vi "init.vi"(8 "error in":errorcluster, 10 "TBM module configuration in":refnum<class "TBM module configuration.lvclass">, 11 "Tag Bus Web Interface runtime in":refnum<class "Tag Bus Web Interface runtime.lvclass">) -> (0 "error out":errorcluster, 1 "data allocations":T1, 2 "execution settings":T4, 3 "Tag Bus Web Interface runtime out":refnum<class "Tag Bus Web Interface runtime.lvclass">)   [LabVIEW 2013, in "Tag Bus Web Interface runtime.lvclass"]
doc: "Provides an interface for initializing a module at runtime. While this interface performs no operations, a child should provide an override which may open any necessary references or sessions, allocate necessary memory, and perform any final configuration validataion before providing the full configuration <b>execution data</b> to the calling process."
uses:
  Tag Bus Web Interface runtime.lvclass
  <vilib>/NI/Tag Bus Module Framework/module configuration/TBM module configuration.lvclass
  <vilib>/NI/Tag Bus Module Framework/runtime/execution settings.ctl
  <vilib>/NI/Tag Bus Module Framework/channel/data tables.ctl
  <vilib>/NI/Tag Bus/dictionary/data dictionary.lvclass
  <vilib>/NI/Tag Bus/dictionary table pair.ctl
  <vilib>/NI/Tag Bus/table/data table.ctl
  configuration/Tag Bus Web Interface configuration.lvclass
  Tag Bus Web Interface runtime.lvclass/Tag Bus Web Interface runtime.ctl
  <vilib>/NI/Tag Bus Module Framework/channel/TBM channel.lvclass
  <vilib>/NI/Tag Bus Module Framework/runtime/TBM module execution interface.lvclass
  <vilib>/NI/Tag Bus/tag bus.lvlib
  <vilib>/NI/Tag Bus/table/data table.lvlib
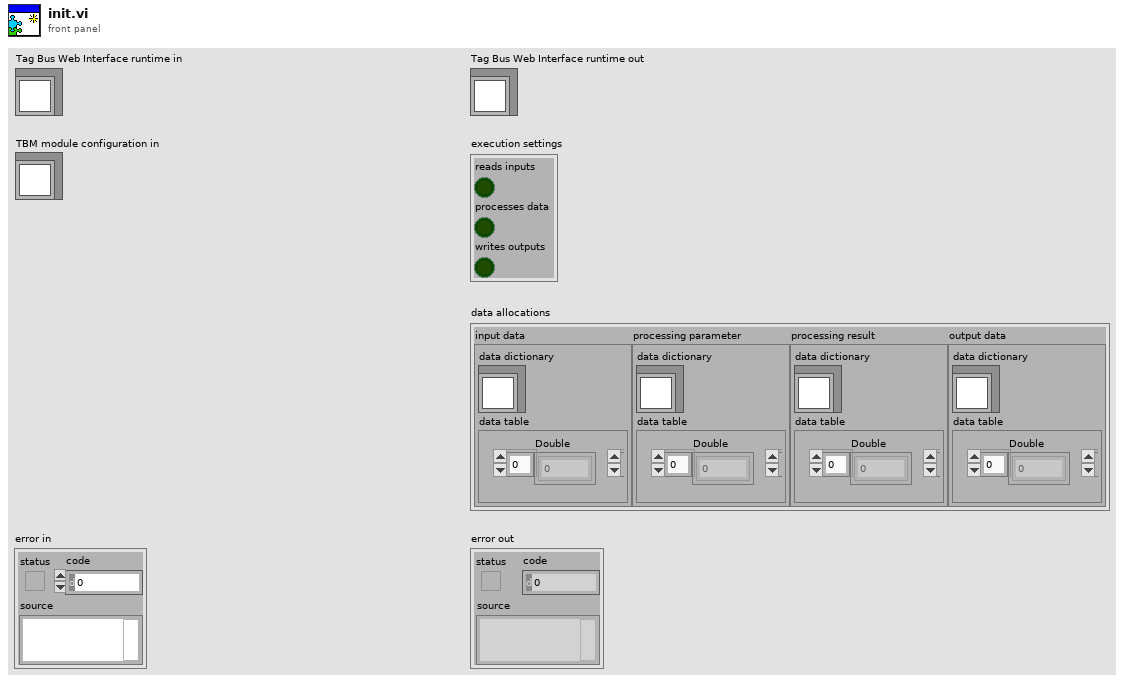
[diagram p1: front panel]
types:
  T1 = typedef "TBM channel.lvclass/data tables.ctl" = cluster{"input data":T2, "processing parameter":T2, "processing result":T2, "output data":T2}
  T2 = typedef "tag bus.lvlib/dictionary table pair.ctl" = cluster{"data dictionary":refnum<class "data dictionary.lvclass">, "data table":T3}
  T3 = typedef "tag bus.lvlib/data table.lvlib/data table.ctl" = cluster{"Double":dbl[], "Single":sgl[], "I64":i64[], "I32":i32[], "I16":i16[], "I8":i8[], "U64":u64[], "U32":u32[], "U16":u16[], "U8":u8[], "Boolean":bool[], "String":string[], "Array of Double":cluster{"DBL Array":dbl[]}[], "Array of Single":cluster{"SGL Array":sgl[]}[], "Array of I64":cluster{"I64 Array":i64[]}[], "Array of I32":cluster{"I32 Array":i32[]}[], "Array of I16":cluster{"I16 Array":i16[]}[], "Array of I8":cluster{"I8 Array":i8[]}[], "Array of U64":cluster{"U64 Array":u64[]}[], "Array of U32":cluster{"U32 Array":u32[]}[], "Array of U16":cluster{"U16 Array":u16[]}[], "Array of U8":cluster{"U8 Array":u8[]}[], "Array of Boolean":cluster{"Boolean Array":bool[]}[], "Array of String":cluster{"String Array":string[]}[]}
  T4 = typedef "TBM module execution interface.lvclass/execution settings.ctl" = cluster{"reads inputs":bool, "processes data":bool, "writes outputs":bool}
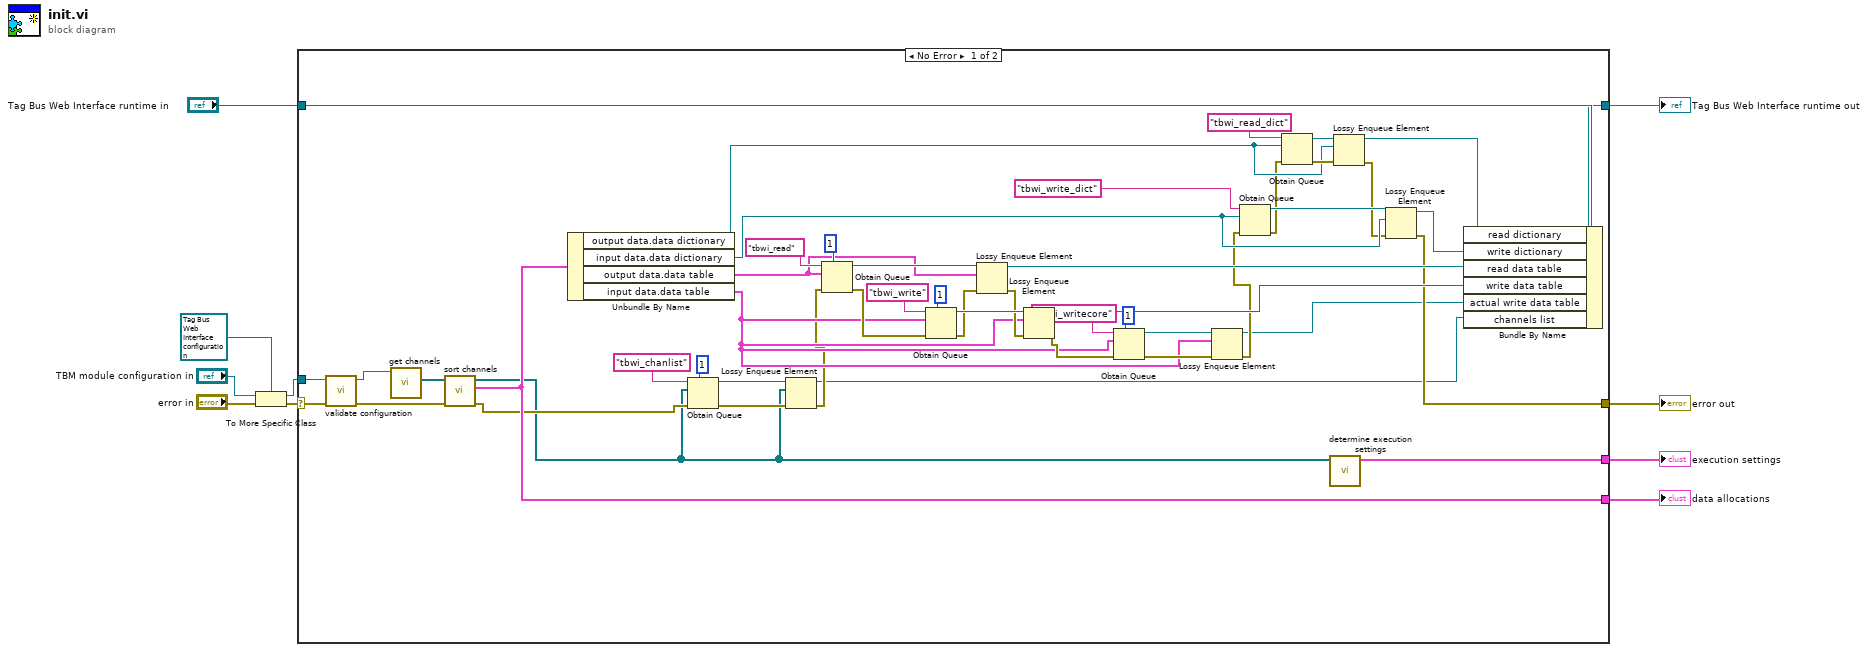
[diagram p0: block diagram]
diagram:
  n1 = To More Specific Class(target class=refnum<class "Tag Bus Web Interface configuration.lvclass"> refnum ("Synchronous module configuration"), reference="TBM module configuration in", error in="error in") -> (specific class reference=w9:refnum<class "Tag Bus Web Interface configuration.lvclass">, error out=w10:errorcluster)
  n2 = case shown="No Error" w10 {
    selector: w10 -> [w57 w60]
    tunnel: w9 -> [w56 _]
    tunnel: "Tag Bus Web Interface runtime in" -> [w29 w61]
    tunnel: [w28 w61] -> w4
    tunnel: [w27 w60] -> w3
    tunnel: [w30 _] -> w1
    tunnel: [w59 _] -> w2
    frame No Error {
      n3 = call-dynamic "validate configuration.vi"("error in"=w57, "Tag Bus Web Interface configuration in"=w56) -> ("error out"=w58:errorcluster, "Tag Bus Web Interface configuration out"=w55:refnum<class "Tag Bus Web Interface configuration.lvclass">)  [unwired: 8 in]
      n4 = call-dynamic "get channels.vi"("Tag Bus Web Interface configuration in"=w55) -> ("channels"=w54:refnum<class "TBM channel.lvclass">[])  [unwired: 9 in, 1 out]
      n5 = call <vilib>:"sort channels.vi"("error in"=w58, "channels in"=w54) -> ("error out"=w14:errorcluster, "data allocations"=w30:T1, "channels out"=w13:refnum<class "TBM channel.lvclass">[])  [unwired: 7 in]
      n6 = Unbundle By Name(w30) -> ("output data.data dictionary"=w40:refnum<class "data dictionary.lvclass">, "input data.data dictionary"=w38:refnum<class "data dictionary.lvclass">, "output data.data table"=w48:T3, "input data.data table"=w20:T3)
      n7 = Obtain Queue(max queue size (-1, unlimited)=1, name (unnamed)="tbwi_chanlist", element data type=w13, error in (no error)=w14) -> (queue out=w17:refnum<queue>, error out=w16:errorcluster)  [unwired: 1 in, 1 out]
      n8 = Lossy Enqueue Element(queue=w17, element=w13, error in (no error)=w16) -> (queue out=w11:refnum<queue>, error out=w12:errorcluster)  [unwired: 2 out]
      n9 = Obtain Queue(max queue size (-1, unlimited)=1, name (unnamed)="tbwi_read", element data type=w48, error in (no error)=w12) -> (queue out=w49:refnum<queue>, error out=w50:errorcluster)  [unwired: 1 in, 1 out]
      n10 = Obtain Queue(max queue size (-1, unlimited)=1, name (unnamed)="tbwi_write", element data type=w20, error in (no error)=w50) -> (queue out=w47:refnum<queue>, error out=w46:errorcluster)  [unwired: 1 in, 1 out]
      n11 = Lossy Enqueue Element(queue=w49, element=w48, error in (no error)=w46) -> (queue out=w33:refnum<queue>, error out=w45:errorcluster)  [unwired: 2 out]
      n12 = Lossy Enqueue Element(queue=w47, element=w20, error in (no error)=w45) -> (queue out=w32:refnum<queue>, error out=w22:errorcluster)  [unwired: 2 out]
      n13 = Obtain Queue(max queue size (-1, unlimited)=1, name (unnamed)="tbwi_writecore", element data type=w20, error in (no error)=w22) -> (queue out=w24:refnum<queue>, error out=w25:errorcluster)  [unwired: 1 in, 1 out]
      n14 = Lossy Enqueue Element(queue=w24, element=w20, error in (no error)=w25) -> (queue out=w19:refnum<queue>, error out=w21:errorcluster)  [unwired: 2 out]
      n15 = Obtain Queue(name (unnamed)="tbwi_write_dict", element data type=w38, error in (no error)=w21) -> (queue out=w39:refnum<queue>, error out=w37:errorcluster)  [unwired: 2 in, 1 out]
      n16 = Obtain Queue(name (unnamed)="tbwi_read_dict", element data type=w40, error in (no error)=w37) -> (queue out=w41:refnum<queue>, error out=w42:errorcluster)  [unwired: 2 in, 1 out]
      n17 = call <vilib>:"determine execution settings.vi"("channels"=w13) -> ("execution settings"=w59:T4)  [unwired: 10 in]
      n18 = Lossy Enqueue Element(queue=w41, element=w40, error in (no error)=w42) -> (queue out=w35:refnum<queue>, error out=w36:errorcluster)  [unwired: 2 out]
      n19 = Lossy Enqueue Element(queue=w39, element=w38, error in (no error)=w36) -> (queue out=w34:refnum<queue>, error out=w27:errorcluster)  [unwired: 2 out]
      n20 = Bundle By Name(cluster=w29, "read dictionary"=w35, "write dictionary"=w34, "read data table"=w33, "write data table"=w32, "actual write data table"=w19, "channels list"=w11) -> (w28:refnum<class "Tag Bus Web Interface runtime.lvclass">)
    }
    frame Error {
    }
  }
  "error out" <- w3
  "Tag Bus Web Interface runtime out" <- w4
  "execution settings" <- w2
  "data allocations" <- w1
